vi "624FastTalonSend.vi"(9 "Data to Send":T1 {"Feedback Select" items=["Digital Quadrature Encoder"=0, "Analog Pot"=2, "Analog Encoder"=3, "Count on Quad-A (Rising-Edge)"=4, "Count on Quad-A (Falling-Edge)"=5, "Position is Pulse-Width"=8]}, 11 "Device ID (0)":u8) -> (0 "error out":errorcluster)   [LabVIEW 2014]
uses:
  <vilib>/Rock Robotics/WPI/CAN/TalonSRX/WPI_CANTalonSRX_GlobalControl.ctl
  <vilib>/Rock Robotics/WPI/CAN/TalonSRX/WPI_CANTalonSRX_APIControlMode.ctl
  <vilib>/Rock Robotics/WPI/CAN/TalonSRX/WPI_CANTalonSRX_BrakeOverride.ctl
  <vilib>/Rock Robotics/WPI/CAN/TalonSRX/WPI_CANTalonSRX_FeedbackSelect.ctl
  <vilib>/Rock Robotics/WPI/CAN/TalonSRX/WPI_CANTalonSRX_MessageIDs.ctl
  <vilib>/Rock Robotics/WPI/CAN/TalonSRX/WPI_CANTalonSRX_ControlMode.ctl
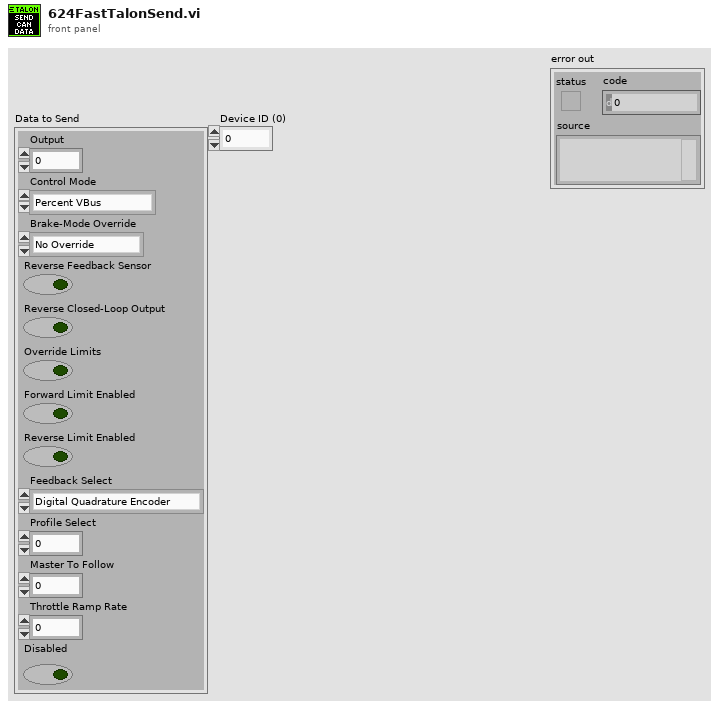
[diagram p1: front panel]
types:
  T1 = typedef "WPI_CANTalonSRX_GlobalControl.ctl" = cluster{"Output":dbl, "Control Mode":T2, "Brake-Mode Override":T3, "Reverse Feedback Sensor":bool, "Reverse Closed-Loop Output":bool, "Override Limits":bool, "Forward Limit Enabled":bool, "Reverse Limit Enabled":bool, "Feedback Select":T4, "Profile Select":u8, "Master To Follow":u8, "Throttle Ramp Rate":u8, "Disabled":bool}
  T2 = typedef "WPI_CANTalonSRX_APIControlMode.ctl" = enum8{"Percent VBus", "Speed", "Position", "Slave", "Unchanged / Invalid"}
  T3 = typedef "WPI_CANTalonSRX_BrakeOverride.ctl" = enum8{"No Override", "Override to Coast", "Override to Brake"}
  T4 = typedef "WPI_CANTalonSRX_FeedbackSelect.ctl" = u8
  T5 = typedef "WPI_CANTalonSRX_MessageIDs.ctl" = u32
  T6 = typedef "WPI_CANTalonSRX_ControlMode.ctl" = enum16{"Throttle (Duty-Cycle)", "Position Closed-Loop", "Velocity Closed-Loop", "Current Closed-Loop", "Voltage Compensation", "Slave Follower"}
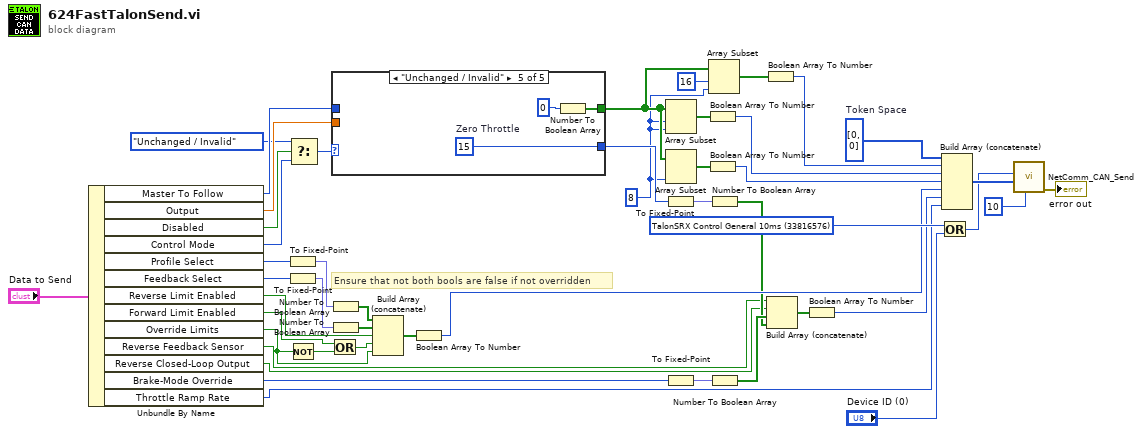
[diagram p0: block diagram]
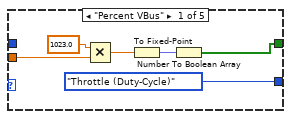
[diagram p2: hidden frame]
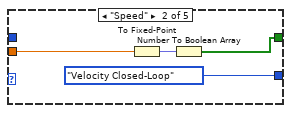
[diagram p3: hidden frame]
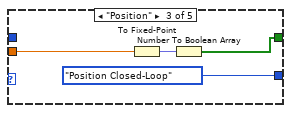
[diagram p4: hidden frame]
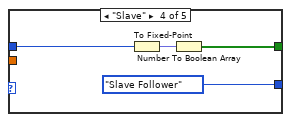
[diagram p5: hidden frame]
diagram:
  w29 = 8 ("length")
  w46 = u8[] [0, 0]  # Token Space
  w45 = T5 33816576 items=["TalonSRX Control General 10ms"=33816576, "TalonSRX Control Rates Slow"=33816640, "TalonSRX Control ClearFlags Slow"=33816704, "TalonSRX Status General 10ms"=33821696, "TalonSRX Status Feedback 20ms"=33821760, "TalonSRX Status Enc 100ms"=33821824, "TalonSRX Status AinTempVbat 100ms"=33821888, "TalonSRX Status Startup Once"=33821952, "TalonSRX Status Debug"=33822080, "TalonSRX Config SetGainsSlot0 A"=33823808, "TalonSRX Config SetGainsSlot0 B"=33823872, "TalonSRX Config SetGainsSlot1 A"=33823936, "TalonSRX Config SetGainsSlot1 B"=33824000, "TalonSRX Config SetSoftLimits"=33824064, "TalonSRX Config WebControl"=33824128, "TalonSRX Param Request"=33822720, "TalonSRX Param Response"=33822784, "TalonSRX Param Set"=33822848]
  # "Ensure that not both bools are false if not overridden"
  n1 = Unbundle By Name("Data to Send") -> ("Master To Follow"=w7:u8, "Output"=w41:dbl, "Disabled"=w4:bool, "Control Mode"=w9:T2, "Profile Select"=w14:u8, "Feedback Select"=w13:T4, "Reverse Limit Enabled"=w17:bool, "Forward Limit Enabled"=w18:bool, "Override Limits"=w15:bool, "Reverse Feedback Sensor"=w12:bool, "Reverse Closed-Loop Output"=w11:bool, "Brake-Mode Override"=w10:T3, "Throttle Ramp Rate"=w6:u8)
  n2 = To Fixed-Point(number=w14) -> (fixed-point=w20:fxp<+,1,1>)  [unwired: 1 in]
  n3 = To Fixed-Point(number=w13) -> (fixed-point=w27:fxp<+,4,4>)  [unwired: 1 in]
  n4 = Not(x=w15) -> (.not. x?=w8:bool)
  n5 = Select(t=WPI_CANTalonSRX_APIControlMode."Unchanged / Invalid", s=w4, f=w9) -> (s? t:f=w5:T2)
  n6 = Or(x=w18, y=w8) -> (x .or. y?=w16:bool)
  n7 = Number To Boolean Array(number=w20) -> (Boolean array=w19:bool[])
  n8 = Number To Boolean Array(number=w27) -> (Boolean array=w26:bool[])
  n9 = case shown="\"Unchanged / Invalid\"" w5 {
    tunnel: w41 -> [w53 w57 w61 _ _]
    tunnel: [WPI_CANTalonSRX_ControlMode."Throttle (Duty-Cycle)" WPI_CANTalonSRX_ControlMode."Velocity Closed-Loop" WPI_CANTalonSRX_ControlMode."Position Closed-Loop" WPI_CANTalonSRX_ControlMode."Slave Follower" w66] -> w35
    tunnel: [w51 w55 w59 w64 w68] -> w30
    tunnel: w7 -> [_ _ _ w62 _]
    frame "Percent VBus" {
      n10 = Multiply(x=1023.0 ("y"), y=w53) -> (x*y=w49:dbl)
      n11 = To Fixed-Point(number=w49) -> (fixed-point=w48:fxp<+/-,24,24>)  [unwired: 1 in]
      n12 = Number To Boolean Array(number=w48) -> (Boolean array=w51:bool[])
    }
    frame "Speed" {
      n13 = To Fixed-Point(number=w57) -> (fixed-point=w54:fxp<+/-,24,24>)  [unwired: 1 in]
      n14 = Number To Boolean Array(number=w54) -> (Boolean array=w55:bool[])
    }
    frame "Position" {
      n15 = To Fixed-Point(number=w61) -> (fixed-point=w58:fxp<+/-,24,24>)  [unwired: 1 in]
      n16 = Number To Boolean Array(number=w58) -> (Boolean array=w59:bool[])
    }
    frame "Slave" {
      n17 = To Fixed-Point(number=w62) -> (fixed-point=w63:fxp<+,6,6>)  [unwired: 1 in]
      n18 = Number To Boolean Array(number=w63) -> (Boolean array=w64:bool[])
    }
    frame "Unchanged / Invalid" {
      w66 = 15  # Zero Throttle
      n19 = Number To Boolean Array(number=0 ("index")) -> (Boolean array=w68:bool[])
    }
  }
  n20 = Build Array (concatenate)(w19, w26, w17, w16, w15) -> (w25:bool[])
  n21 = Boolean Array To Number(Boolean array=w25) -> (number=w24:u32)
  n22 = Array Subset(array=w30, index=w29, length=w29) -> (w33:bool[])
  n23 = Array Subset(array=w30, length=w29) -> (w32:bool[])  [unwired: 1 in]
  n24 = To Fixed-Point(number=w35) -> (fixed-point=w36:fxp<+,4,4>)  [unwired: 1 in]
  n25 = To Fixed-Point(number=w10) -> (fixed-point=w23:fxp<+,2,2>)  [unwired: 1 in]
  n26 = Boolean Array To Number(Boolean array=w33) -> (number=w39:u32)
  n27 = Boolean Array To Number(Boolean array=w32) -> (number=w38:u32)
  n28 = Array Subset(array=w30, index=16, length=w29) -> (w31:bool[])
  n29 = Number To Boolean Array(number=w36) -> (Boolean array=w21:bool[])
  n30 = Number To Boolean Array(number=w23) -> (Boolean array=w22:bool[])
  n31 = Boolean Array To Number(Boolean array=w31) -> (number=w34:u32)
  n32 = Build Array (concatenate)(w12, w11, w22, w21) -> (w37:bool[])
  n33 = Boolean Array To Number(Boolean array=w37) -> (number=w40:u32)
  n34 = Or(x=w45, y="Device ID (0)") -> (x .or. y?=w44:T5)
  n35 = Build Array (concatenate)(w46, w34, w39, w38, w24, w40, w6) -> (w47:u32[])
  n36 = call <vilib>:"NetComm_CAN_Send.vi"("Period (ms)"=10 ("milliseconds to wait"), "Data"=w47, "Message ID"=w44) -> ("error out"=→"error out":errorcluster)  [unwired: 8 in]
